vi "BuildTagArray.vi"(0 "Indent":i8=-1, 2 "tags":string[](array[string]), 3 "value":string, 4 "string in":string) -> (1 "string out":string)   [LabVIEW 2018]
doc: "Encloses the value in the array of tags. Appends the value to string in"
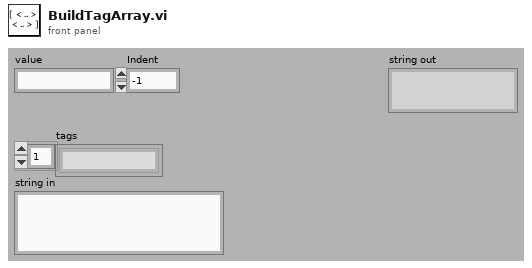
[diagram p1: front panel]
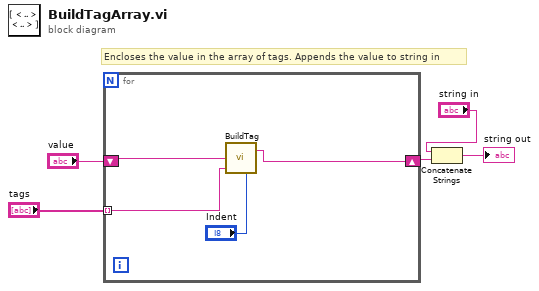
[diagram p0: block diagram]
diagram:
  # "Encloses the value in the array of tags. Appends the value to string in"
  n1 = for {
    shift-right: [w8] -> w3
    shift-left: "value" -> [w9]
    tunnel: "tags" -> [w7] mode=indexing
    n2 = call <userlib>:"BuildTag.vi"("Indent"="Indent", "tag"=w7, "value"=w9) -> ("string out"=w8:string)  [unwired: 1 in]
  }
  n3 = Concatenate Strings("string in", w3) -> (→"string out":string)
